vi "Engine Control FPGA.vi"() -> ()   [LabVIEW 2015]
uses:
  <vilib>/Platform/TimedLoop/XDataNode/timing_clust.ctl
  <vilib>/Platform/TimedLoop/XDataNode/nitl_modes.ctl
  <vilib>/Platform/TimedLoop/XDataNode/wakeup.ctl
  <vilib>/rvi/Emulation/niFpgaSctlEmulationGetInTimedLoop.vi
  <vilib>/rvi/Emulation/niFpgaEmulationReportErrorSimple.vi
  <vilib>/rvi/Emulation/niFpgaGetClockAttributes.vi
  <vilib>/rvi/Emulation/niFpgaCriticalErrorInLSC.vi
  <vilib>/Platform/TimedLoop/XDataNode/XDataNode.xnode
  <vilib>/Platform/TimedLoop/XDataNode/XDNodeRunTimeDep.lvlib
panel:
  in  "FuelControl":T1
  in  "SparkControl":T2
  in  "MPControl1":T3
  in  "MPControl2":T4
  in  "MPControl3":T5
  in  "MPControl4":T6
  in  "PFIControl":T7
  in  "LowsidePWM":T8
  out "PFIData":T9
  in  "FuelControl1":T1
  in  "FuelControl2":T1
  in  "PFI_IPhaseInterface":T10(array[cluster])=[{"IPhaseCurrent"=0, "IPhaseDuration"=0}, {"IPhaseCurrent"=0, "IPhaseDuration"=0}, {"IPhaseCurrent"=0, "IPhaseDuration"=0}, {"IPhaseCurrent"=0, "IPhaseDuration"=0}, {"IPhaseCurrent"=0, "IPhaseDuration"=0}, {"IPhaseCurrent"=0, "IPhaseDuration"=0}, {"IPhaseCurrent"=0, "IPhaseDuration"=0}, {"IPhaseCurrent"=0, "IPhaseDuration"=0}] caption="IPhaseInterface"
  in  "DI1_ScopeRead":bool caption="DIScopeRead"
  in  "EPTControl":T11
  in  "DI1_IPhaseInterface":T12(array[cluster]) caption="IPhaseInterface"
  in  "DI1_Control":T13 caption="DIControl"
  out "DI1_ScopeData":T14 caption="DIScopeData"
  in  "PlsGen_Config_Channel1":T15
  out "EPTData":T16
  out "DI1_Data":T17 caption="DIData"
  # "PFI"
  # "EPT"
  # "DI"
  # "Spark"
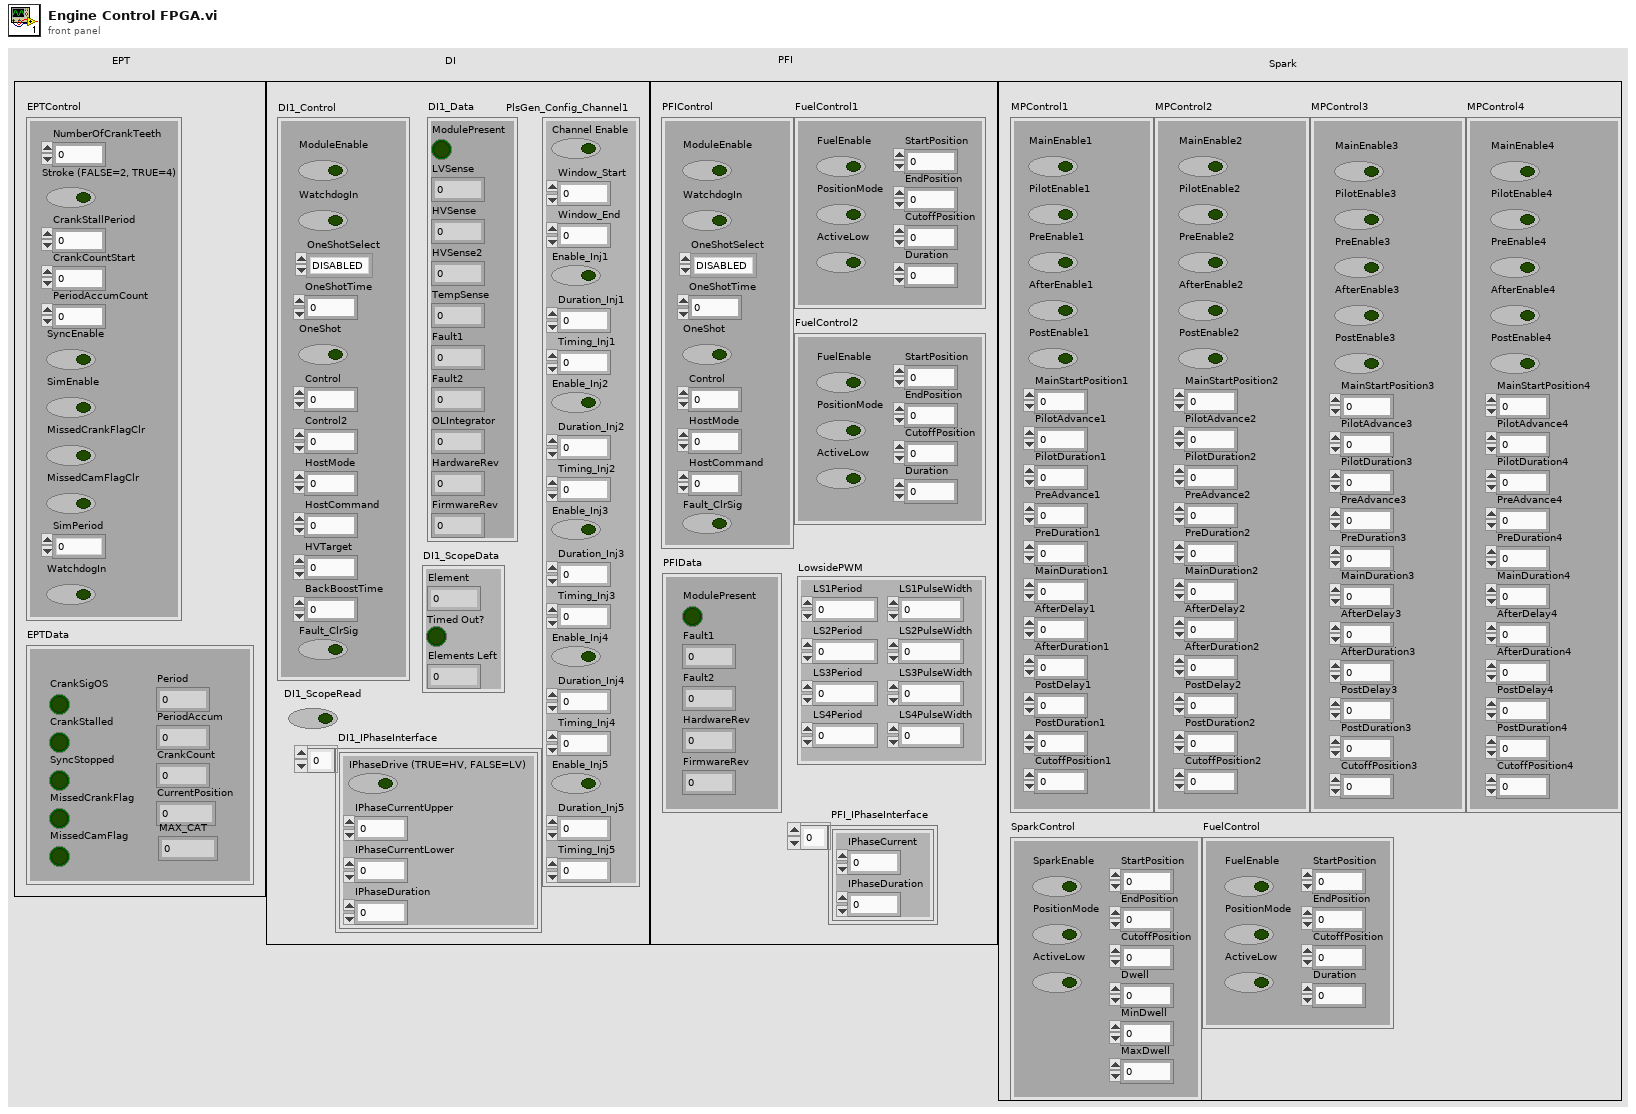
[diagram p1: front panel]
types:
  T1 = cluster{"FuelEnable":bool, "PositionMode":bool, "ActiveLow":bool, "StartPosition":u16, "EndPosition":u16, "CutoffPosition":u16, "Duration":u32}
  T2 = cluster{"SparkEnable":bool, "PositionMode":bool, "ActiveLow":bool, "StartPosition":u16, "EndPosition":u16, "CutoffPosition":u16, "Dwell":u32, "MinDwell":u32, "MaxDwell":u32}
  T3 = cluster{"MainEnable1":bool, "PilotEnable1":bool, "PreEnable1":bool, "AfterEnable1":bool, "PostEnable1":bool, "MainStartPosition1":u16, "PilotAdvance1":u32, "PilotDuration1":u32, "PreAdvance1":u32, "PreDuration1":u32, "MainDuration1":u32, "AfterDelay1":u32, "AfterDuration1":u32, "PostDelay1":u32, "PostDuration1":u32, "CutoffPosition1":u16}
  T4 = cluster{"MainEnable2":bool, "PilotEnable2":bool, "PreEnable2":bool, "AfterEnable2":bool, "PostEnable2":bool, "MainStartPosition2":u16, "PilotAdvance2":u32, "PilotDuration2":u32, "PreAdvance2":u32, "PreDuration2":u32, "MainDuration2":u32, "AfterDelay2":u32, "AfterDuration2":u32, "PostDelay2":u32, "PostDuration2":u32, "CutoffPosition2":u16}
  T5 = cluster{"MainEnable3":bool, "PilotEnable3":bool, "PreEnable3":bool, "AfterEnable3":bool, "PostEnable3":bool, "MainStartPosition3":u16, "PilotAdvance3":u32, "PilotDuration3":u32, "PreAdvance3":u32, "PreDuration3":u32, "MainDuration3":u32, "AfterDelay3":u32, "AfterDuration3":u32, "PostDelay3":u32, "PostDuration3":u32, "CutoffPosition3":u16}
  T6 = cluster{"MainEnable4":bool, "PilotEnable4":bool, "PreEnable4":bool, "AfterEnable4":bool, "PostEnable4":bool, "MainStartPosition4":u16, "PilotAdvance4":u32, "PilotDuration4":u32, "PreAdvance4":u32, "PreDuration4":u32, "MainDuration4":u32, "AfterDelay4":u32, "AfterDuration4":u32, "PostDelay4":u32, "PostDuration4":u32, "CutoffPosition4":u16}
  T7 = cluster{"ModuleEnable":bool, "WatchdogIn":bool, "OneShotSelect":enum8{"DISABLED", "PFI 1", "PFI 2", "PFI 3", "PFI 4"}, "OneShotTime":u32, "OneShot":bool, "Control":u16, "HostMode":u8, "HostCommand":u32, "Fault_ClrSig":bool}
  T8 = cluster{"LS1Period":u32, "LS1PulseWidth":u32, "LS2Period":u32, "LS2PulseWidth":u32, "LS3Period":u32, "LS3PulseWidth":u32, "LS4Period":u32, "LS4PulseWidth":u32}
  T9 = cluster{"ModulePresent":bool, "Fault1":u8, "Fault2":u8, "HardwareRev":u8, "FirmwareRev":u8}
  T10 = cluster{"IPhaseCurrent":u16, "IPhaseDuration":u16}[]
  T11 = cluster{"NumberOfCrankTeeth":u16, "Stroke (FALSE=2, TRUE=4)":bool, "CrankStallPeriod":u32, "CrankCountStart":u16, "PeriodAccumCount":u16, "SyncEnable":bool, "SimEnable":bool, "MissedCrankFlagClr":bool, "MissedCamFlagClr":bool, "SimPeriod":u32, "WatchdogIn":bool}
  T12 = cluster{"IPhaseDrive (TRUE=HV, FALSE=LV)":bool, "IPhaseCurrentUpper":u16, "IPhaseCurrentLower":u16, "IPhaseDuration":u16}[]
  T13 = cluster{"ModuleEnable":bool, "WatchdogIn":bool, "OneShotSelect":enum8{"DISABLED", "CHAN 1", "CHAN 2", "CHAN 3"}, "OneShotTime":u32, "OneShot":bool, "Control":u8, "Control2":u8, "HostMode":u8, "HostCommand":u32, "HVTarget":u8, "BackBoostTime":u8, "Fault_ClrSig":bool}
  T14 = cluster{"Element":u32, "Timed Out?":bool, "Elements Left":u32}
  T15 = cluster{"Channel Enable":bool, "Window_Start":u16, "Window_End":u16, "Enable_Inj1":bool, "Duration_Inj1":u32, "Timing_Inj1":u16, "Enable_Inj2":bool, "Duration_Inj2":u32, "Timing_Inj2":u16, "Enable_Inj3":bool, "Duration_Inj3":u32, "Timing_Inj3":u16, "Enable_Inj4":bool, "Duration_Inj4":u32, "Timing_Inj4":u16, "Enable_Inj5":bool, "Duration_Inj5":u32, "Timing_Inj5":u16}
  T16 = cluster{"CrankSigOS":bool, "CrankStalled":bool, "SyncStopped":bool, "MissedCrankFlag":bool, "MissedCamFlag":bool, "Period":u32, "PeriodAccum":u32, "CrankCount":u16, "CurrentPosition":u16, "MAX_CAT":u16}
  T17 = cluster{"ModulePresent":bool, "LVSense":u8, "HVSense":u8, "HVSense2":u8, "TempSense":i8, "Fault1":u8, "Fault2":u8, "OLIntegrator":u32, "HardwareRev":u8, "FirmwareRev":u8}
  T18 = typedef "XDNodeRunTimeDep.lvlib/timing_clust.ctl" = cluster{"Expected End [f-1]":u64, "Actual End [f-1]":u64, "Finished Late? [f-1]":bool, "Expected End [i-1]":u64, "Actual End [i-1]":u64, "Finished Late? [i-1]":bool, "Expected Start [i]":u64, "Actual Start [i]":u64, "Expected Start [f]":u64, "Actual Start [f]":u64, "Source Name":string, "Structure Name":string, "Period":i64, "Deadline":i64, "Offset":i64, "Start":i64, "Priority":i32, "Timeout":i32, "Mode":T19, "Wakeup Reason":T20, "Error":errorcluster, "Source Type":string, "Secondary Source Type":string, "Global End Time":u64, "Global Start Time":u64, "Frame Duration":u64, "Iteration Duration":u64, "Assigned CPU":i32, "I/O Scan Engine Mode":u32}
  T19 = typedef "XDNodeRunTimeDep.lvlib/nitl_modes.ctl" = enum32{"No Change", "Process missed periods, maintain original phase", "Discard missed periods, maintain original phase", "Process missed periods, ignore original phase", "Discard missed periods, ignore original phase"}
  T20 = typedef "XDNodeRunTimeDep.lvlib/wakeup.ctl" = enum32{"Normal", "Aborted", "Asynchronous wakeup", "Timing source error", "Timed loop error", "Timeout"}
  T21 = cluster{"FSSup0":bool, "FSSup1":bool, "FSSup2":bool, "FSSup3":u16, "FSSup4":u32, "FSSup5":u16}
  T22 = cluster{"FIOut":bool, "SparkOut":bool, "CrankSigOut":bool, "CamSigOut":bool, "MPOut1":bool, "MPOut2":bool, "MPOut3":bool, "MPOut4":bool}
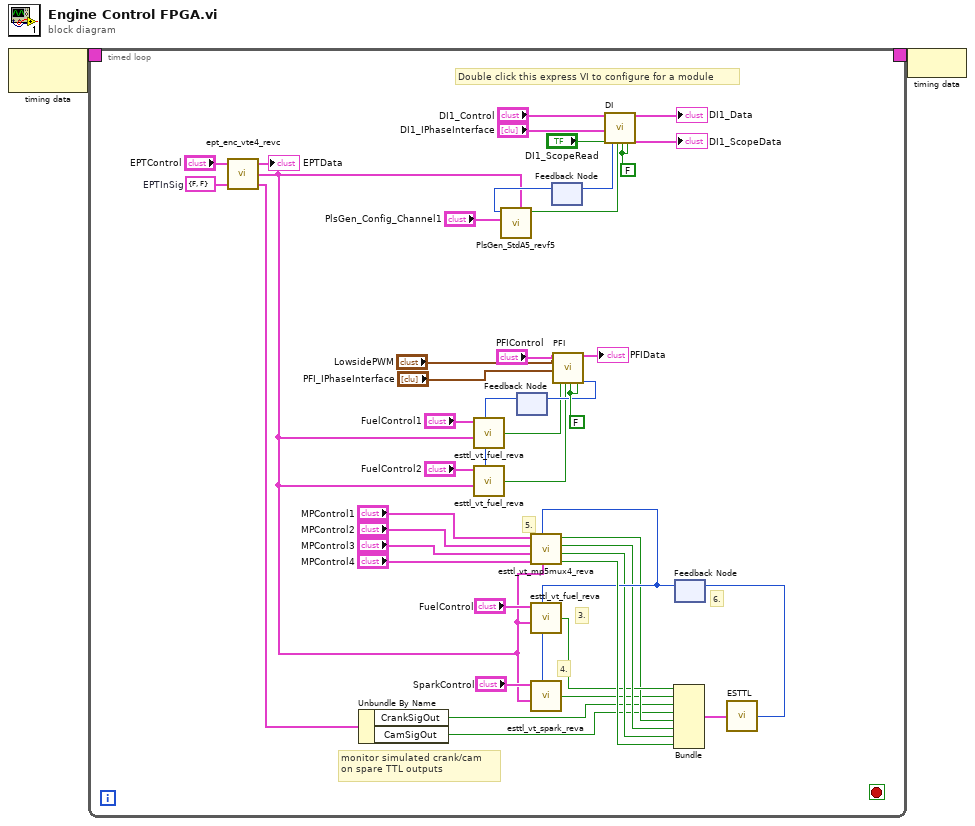
[diagram p0: block diagram]
diagram:
  n1 = node-c288() -> (w2:T18)  [unwired: 1 in]
  n2 = timed-loop {
    timing: w2 -> [_]
    timing-out: [_] -> w1
    stop <- _ stop-if-true
    w32 = FALSE ("PFI3Cmd")
    w33 = FALSE ("DI2Cmd")
    w44 = cluster{"CrankSig":bool, "CamSig":bool} {"CrankSig"=FALSE, "CamSig"=FALSE}  # EPTInSig
    # "6."
    # "5."
    # "4."
    # "3."
    # "monitor simulated crank/cam\non spare TTL outputs"
    # "Double click this express VI to configure for a module"
    n3 = call <vilib>:"ept_enc_vte4_revc.vi"("EPTControl"="EPTControl", "EPTInSig"=w44) -> ("EPTData"=→"EPTData":T16, "FuelSparkSupervisor"=w4:T21, "EPTOutSig"=w3:cluster{"CrankSigOut":bool, "CamSigOut":bool})  [unwired: 3 in]
    n4 = Unbundle By Name(w3) -> ("CrankSigOut"=w8:bool, "CamSigOut"=w9:bool)
    n5 = feedback #1() -> (w24:u16)  [unwired: 1 in]
    n6 = call <vilib>:"esttl_vt_fuel_reva.vi"("FuelControl"="FuelControl1", "Key"=w24, "FuelSparkSupervisor"=w4) -> ("FIOut"=w29:bool)  [unwired: 5 in]
    n7 = call <vilib>:"esttl_vt_fuel_reva.vi"("FuelControl"="FuelControl2", "Key"=w24, "FuelSparkSupervisor"=w4) -> ("FIOut"=w30:bool)  [unwired: 5 in]
    n8 = feedback #2() -> (w35:u16)  [unwired: 1 in]
    n9 = call <vilib>:"PlsGen_StdA5_revf5.vi"("PlsGen_Config_Channel1"="PlsGen_Config_Channel1", "key"=w35, "FuelSparkSupervisor"=w4) -> ("CmdOut1"=w34:bool)  [unwired: 4 in, 2 out]
    n10 = call "PFI"("PFIControl"="PFIControl", "LowsidePWM"="LowsidePWM", "PFIIPhaseArray"="PFI_IPhaseInterface", "PFI1Cmd"=w29, "PFI2Cmd"=w30, "PFI3Cmd"=w32, "PFI4Cmd"=w32) -> ("PFIData"=→"PFIData":T9, "Key Out"=w31:u16)  [unwired: 11 in]
    n11 = feedback-in #1(w31) -> ()
    n12 = call "DI"("DIControl"="DI1_Control", "IPhaseInterface"="DI1_IPhaseInterface", "DIScopeRead"="DI1_ScopeRead", "DI1Cmd"=w34, "DI2Cmd"=w33, "DI3Cmd"=w33) -> ("Key Out"=w36:u16, "DIData"=→"DI1_Data":T17, "DIScopeData"=→"DI1_ScopeData":T14)  [unwired: 11 in]
    n13 = feedback-in #2(w36) -> ()
    n14 = feedback #3() -> (w19:u16)  [unwired: 1 out]
    n15 = call <vilib>:"esttl_vt_mp5mux4_reva.vi"("FuelSparkSupervisor"=w4, "Key"=w19, "MPControl4"="MPControl4", "MPControl3"="MPControl3", "MPControl2"="MPControl2", "MPControl1"="MPControl1") -> ("MPOut4"=w20:bool, "MPOut3"=w18:bool, "MPOut2"=w17:bool, "MPOut1"=w11:bool)  [unwired: 2 out]
    n16 = call <vilib>:"esttl_vt_fuel_reva.vi"("FuelControl"="FuelControl", "Key"=w19, "FuelSparkSupervisor"=w4) -> ("FIOut"=w16:bool)  [unwired: 5 out]
    n17 = call <vilib>:"esttl_vt_spark_reva.vi"("SparkControl"="SparkControl", "Key"=w19, "FuelSparkSupervisor"=w4) -> ("SparkOut"=w10:bool)  [unwired: 5 out]
    n18 = Bundle("FIOut"=w16, "SparkOut"=w10, "CrankSigOut"=w8, "CamSigOut"=w9, "MPOut1"=w11, "MPOut2"=w17, "MPOut3"=w18, "MPOut4"=w20) -> (w21:T22)  [unwired: 1 out]
    n19 = call "ESTTL"("ESTTLChan"=w21) -> ("Key"=w7:u16)
    n20 = feedback-in #3(w7) -> ()
  }
  n21 = node-c288(w1) -> ()
